vi "cos_gen.vi"(2 "Seno/Coseno":bool, 3 "Cantidad de muestras":i32=10000, 4 "Frecuencia de muestreo":dbl=1000.0, 5 "Frecuencia":dbl=1.0) -> (0 "Salida Sobremuestreada":waveform(dbl), 1 "Salida":waveform(dbl))   [LabVIEW 2018]
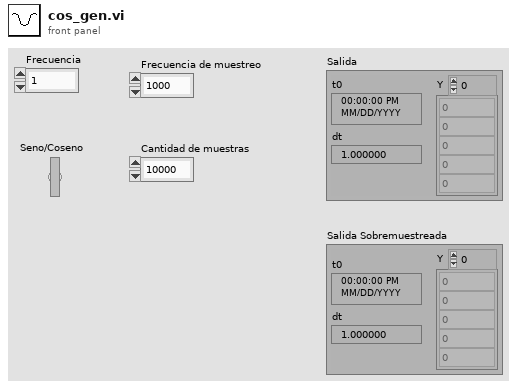
[diagram p1: front panel]
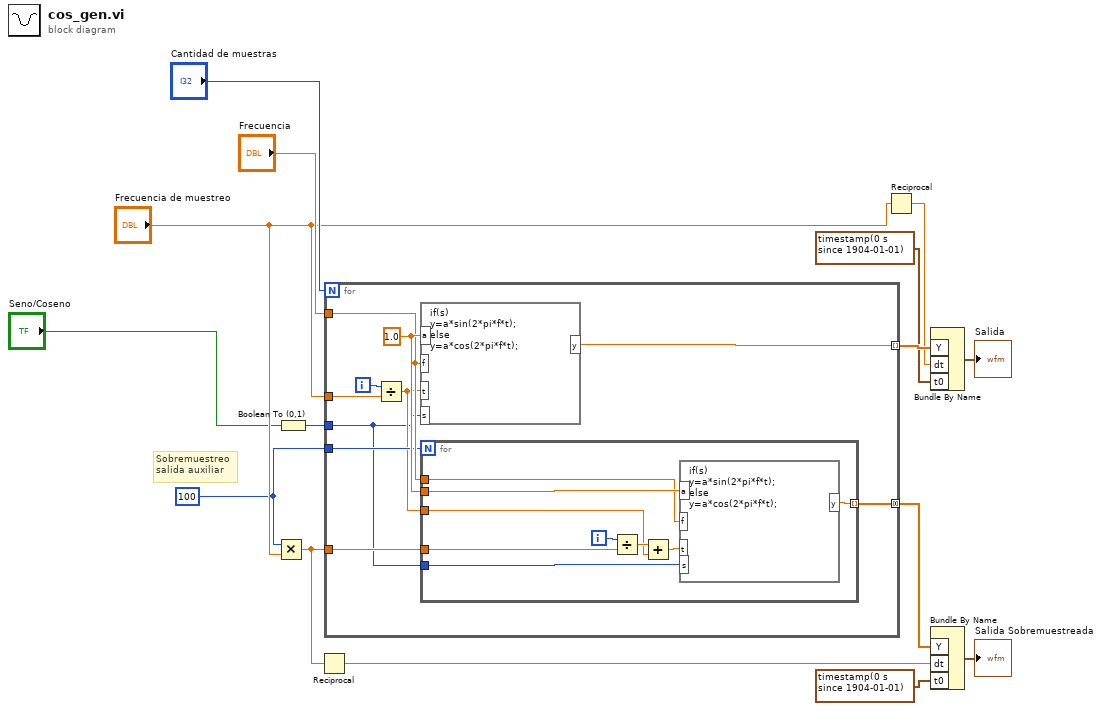
[diagram p0: block diagram]
diagram:
  w3 = 100
  # "Sobremuestreo\nsalida auxiliar"
  n1 = Multiply(x=w3, y="Frecuencia de muestreo") -> (x*y=w7:dbl)
  n2 = Boolean To (0,1)(Boolean="Seno/Coseno") -> (0, 1=w1:i16)
  n3 = Reciprocal(x=w7) -> (1/x=w10:dbl)
  n4 = for {
    N: "Cantidad de muestras" -> [_]
    tunnel: "Frecuencia" -> [w24]
    tunnel: w3 -> [w23]
    tunnel: "Frecuencia de muestreo" -> [w22]
    tunnel: [w19] -> w13 mode=indexing
    tunnel: w7 -> [w18]
    tunnel: [w17] -> w6 mode=concatenating
    tunnel: w1 -> [w16]
    i -> [w21]
    w25 = 1.0 ("input variable")
    n5 = Divide(x=w21, y=w22) -> (x/y=w20:dbl)
    n6 = formula code="if(s)\ny=a*sin(2*pi*f*t);\nelse\ny=a*cos(2*pi*f*t);"("a"=w25, "f"=w24, "t"=w20, "s"=w16) -> ("y"=w19:dbl)
    n7 = for {
      N: w23 -> [_]
      tunnel: w25 -> [w34]
      tunnel: w24 -> [w33]
      tunnel: w18 -> [w32]
      tunnel: w20 -> [w29]
      tunnel: [w27] -> w17 mode=indexing
      tunnel: w16 -> [w26]
      i -> [w31]
      n8 = Divide(x=w31, y=w32) -> (x/y=w30:dbl)
      n9 = Add(x=w30, y=w29) -> (x+y=w28:dbl)
      n10 = formula code="if(s)\ny=a*sin(2*pi*f*t);\nelse\ny=a*cos(2*pi*f*t);"("a"=w34, "f"=w33, "t"=w28, "s"=w26) -> ("y"=w27:dbl)
    }
  }
  n11 = Reciprocal(x="Frecuencia de muestreo") -> (1/x=w9:dbl)
  n12 = Bundle By Name("Y"=w13, "dt"=w9, "t0"=timestamp(0 s since 1904-01-01)) -> (→"Salida":waveform(dbl))  [unwired: 1 in]
  n13 = Bundle By Name("Y"=w6, "dt"=w10, "t0"=timestamp(0 s since 1904-01-01)) -> (→"Salida Sobremuestreada":waveform(dbl))  [unwired: 1 in]
